vi "Read Connections.vi"(8 "error in":errorcluster, 11 "CoreOOB_Rx in":refnum<class "CIFCoreOOB_Rx.lvclass">) -> (0 "error out":errorcluster, 1 "Offset":i32, 2 "Connections":T1[](array[typedef]) {"Connection Data" format="%x"}, 3 "CoreOOB_Rx out":refnum<class "CIFCoreOOB_Rx.lvclass">)   [LabVIEW 2021, in "CIFCoreOOB_Rx.lvclass"]
uses:
  CIFCoreOOB_Rx.lvclass
  D:/dev/CIF-LVCore/src/CIFUtilities/CIFOutOfBand/CIFOutOfBand.lvclass
  Typedef/Channel Connection Data.ctl
  CIFUtilities/CIFOutOfBand/CIFOutOfBand.lvclass/CIFOutOfBand.ctl
  CIFCoreOOB_Rx.lvclass/CIFCoreOOB_Rx.ctl
  CIFUtilities/CIFOutOfBand/Accessors/Read Local OOB Data.vi
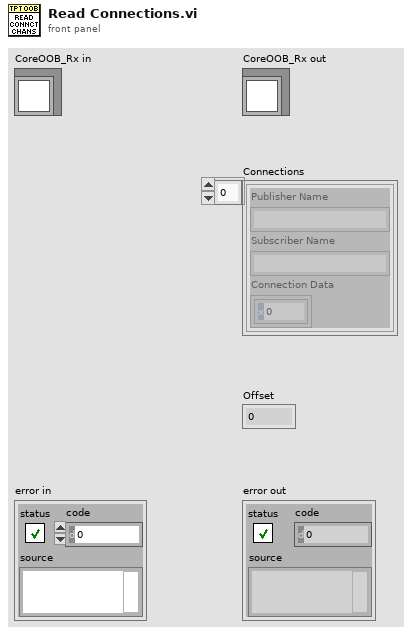
[diagram p1: front panel]
types:
  T1 = typedef "CIFCoreOOB_Rx.lvclass/Channel Connection Data.ctl" = cluster{"Publisher Name":string, "Subscriber Name":string, "Connection Data":u8[]}
  T2 = typedef "CIFCoreOOB_Rx.lvclass/Template Payload.ctl" = cluster{"Config Data":variant, "Connections":T1[]}
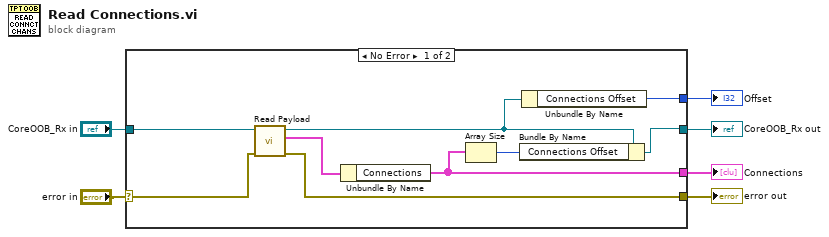
[diagram p0: block diagram]
diagram:
  n1 = case shown="No Error" "error in" {
    selector: "error in" -> [w15 w17]
    tunnel: [w13 w17] -> w6
    tunnel: [w11 w16] -> w5
    tunnel: "CoreOOB_Rx in" -> [w12 w16]
    tunnel: [w8 _] -> w1
    tunnel: [w9 _] -> w2
    frame No Error {
      n2 = call "Read Payload.vi"("error in"=w15, "CoreOOB_Rx in"=w12) -> ("error out"=w13:errorcluster, "data"=w14:T2, "CoreOOB_Rx out"=w10:refnum<class "CIFCoreOOB_Rx.lvclass">)  [unwired: 7 in]
      n3 = Unbundle By Name(w14) -> ("Connections"=w8:T1[])
      n4 = Array Size(array=w8) -> (size(s)=w7:i32)
      n5 = Bundle By Name(cluster=w10, "Connections Offset"=w7) -> (w11:refnum<class "CIFCoreOOB_Rx.lvclass">)
      n6 = Unbundle By Name(w10) -> ("Connections Offset"=w9:i32)
    }
    frame Error {
    }
  }
  "error out" <- w6
  "CoreOOB_Rx out" <- w5
  "Offset" <- w2
  "Connections" <- w1
